vi "libc path.vi"(8 "error in (no error)":errorcluster) -> (0 "error out":errorcluster, 3 "path to libc":path)   [LabVIEW 2013, in "Linux RT IPC.lvlib" / "Shared Memory.lvlib" / "Shared Memory.lvclass"]
doc: "Stores path to standard c library (glibc)."
uses:
  Shared Memory.lvclass
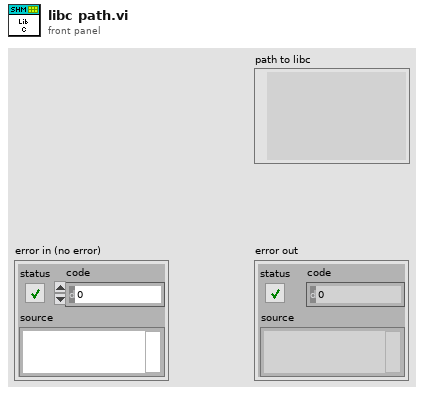
[diagram p1: front panel]
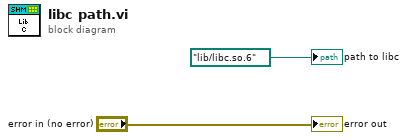
[diagram p0: block diagram]
diagram:
  "error out" <- "error in (no error)"
  "path to libc" <- path "/lib/libc.so.6" ("path to libc")
